vi "Ubidots_POST.vi"() -> ()   [LabVIEW 2013]
uses:
  <vilib>/httpClient/POSTBuffer.vi
  <vilib>/httpClient/LabVIEWHTTPClient.lvlib
panel:
  in  "Value to Send":string
  in  "Auth Token":string
  in  "Variable ID":string
  out "POST Response":string
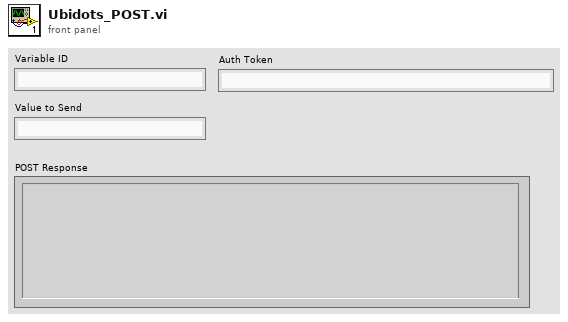
[diagram p1: front panel]
types:
  T1 = typedef "LabVIEWHTTPClient.lvlib/ClientHandle.ctl" = refnum<k1>
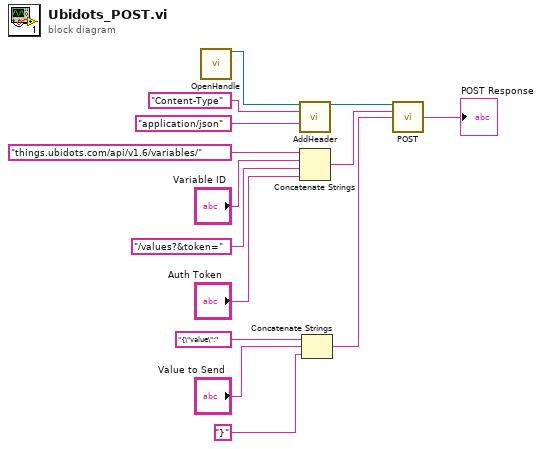
[diagram p0: block diagram]
diagram:
  n1 = call <vilib>:"OpenHandle.vi"() -> ("client handle out"=w5:T1)  [unwired: 14 in, 1 out]
  n2 = call <vilib>:"AddHeader.vi"("client handle"=w5, "header"="Content-Type" ("format string"), "value"="application/json" ("format string")) -> ("client handle out"=w8:T1)  [unwired: 11 in, 1 out]
  n3 = Concatenate Strings("things.ubidots.com/api/v1.6/variables/", "Variable ID", "/values?&token=", "Auth Token") -> (w9:string)
  n4 = Concatenate Strings("{\"value\":" ("format string"), "Value to Send", "}" ("format string")) -> (w1:string)
  n5 = call-poly <vilib>:"POST.vi"("client handle"=w8, "url"=w9, "buffer"=w1) -> ("body"=→"POST Response":string)  [unwired: 9 in, 3 out]
